vi "Memory Location Update.vi"(7 "Memory In":refnum<k21>, 8 "Data Valid":bool=TRUE, 10 "Address":u16, 11 "Data":fxp<+/-,16,1>) -> ()   [LabVIEW 2011]
uses:
  <vilib>/rvi/FXPMathLib/FxpConvert/subVIs/nifxpmath_Convert_SimConfig.ctl
  <vilib>/fxp/LVFixedPointQuantizationPolicyTypeDef.ctl
  <vilib>/fxp/LVFixedPointOverflowPolicyTypeDef.ctl
  <vilib>/rvi/FXPMathLib/basic elements/DSP48E/simVIs/niFpgaDsp48eRegisters.ctl
  <vilib>/rvi/FXPMathLib/basic elements/DSP48E/simVIs/niFpgaDsp48eEnables.ctl
  <vilib>/rvi/FXPMathLib/basic elements/DSP48E/simVIs/niFpgaDsp48eResets.ctl
  <vilib>/rvi/FXPMathLib/basic elements/DSP48E/simVIs/niFpgaDsp48eSimulationState.ctl
  <vilib>/rvi/FXPMathLib/basic elements/DSP48E/subVIs/niFpgaDsp48eType.ctl
  <vilib>/rvi/FXPMathLib/basic elements/DSP48E/subVIs/niFpgaDsp48eAlumodeOpmodeCarryinselState.ctl
  <vilib>/rvi/FXPMathLib/basic elements/DSP48E/subVIs/niFpgaDsp48eUseMultiplierState.ctl
  <vilib>/rvi/FXPMathLib/basic elements/DSP48E/subVIs/niFpgaDsp48eLogicUnitModeState.ctl
  <vilib>/rvi/FXPMathLib/basic elements/DSP48E/subVIs/niFpgaDsp48eSelectPatternState.ctl
  <vilib>/rvi/FXPMathLib/basic elements/DSP48E/subVIs/niFpgaDsp48eSelectMaskState.ctl
  <vilib>/rvi/FXPMathLib/basic elements/DSP48E/subVIs/niFpgaDsp48eAutoresetState.ctl
  <vilib>/rvi/FXPMathLib/FxpConvert/simVIs/DllFxpConvertTemp_sub.vi
  <vilib>/rvi/FXPMathLib/basic elements/DSP48E/simVIs/niFpgaDsp48eSimMultiplier.vi
  <vilib>/rvi/FXPMathLib/basic elements/DSP48E/simVIs/niFpgaDsp48eSimArithmetic.vi
  <vilib>/rvi/FXPMathLib/basic elements/DSP48E/simVIs/niFpgaDsp48eSimPatternDetect.vi
  <vilib>/rvi/FXPMathLib/basic elements/DSP48E/simVIs/niFpgaDsp48eSimP.vi
  <vilib>/rvi/FXPMathLib/basic elements/DSP48E/simVIs/niFpgaDsp48eSimUpdateState.vi
  <vilib>/rvi/FXPMathLib/basic elements/DSP48E/simVIs/niFpgaDsp48eCheckMode.vi
  <vilib>/rvi/FXPMathLib/basic elements/DSP48E/simVIs/niFpgaDsp48eReportInvalidMode.vi
  <vilib>/rvi/DataTransferAndStorage/Container/Common/niFpgaContainerExecOnDevCompGetState.vi
  <vilib>/rvi/Memory/Memory_Emulation/niFpgaMemoryEmulationValidateCache.vi
  <vilib>/rvi/DataTransferAndStorage/Container/Common/niFpgaContainerGetUniqueNameForEmu.vi
  <vilib>/rvi/Memory/Memory_Emulation/nirvimemoryEmulationManagerCache_InsertValue.vi
  <vilib>/Utility/error.llb/Clear Errors.vi
  <vilib>/rvi/Memory/Memory_Emulation/nirvimemoryEmulationManagerCache_GetValue.vi
  <vilib>/rvi/Memory/Memory_Emulation/nirvimemoryEmulationManagerCache_SetValue.vi
  <vilib>/rvi/FXPMathLib/FxpConvert/XNode/nifxpmath_Convert.xnode
  <vilib>/rvi/FXPMathLib/basic elements/DSP48E/XNode/niFpgaDsp48e.xnode
  <vilib>/rvi/FXPMathLib/basic elements/FxpDiscreteDelay/XNode/nifxpmath_DiscreteDelay.xnode
  <vilib>/rvi/DataTransferAndStorage/Container/XNode/niFpgaContainer.xnode
  <vilib>/rvi/Memory/Memory_Emulation/niFpgaMemoryEmulationRefIn.vi
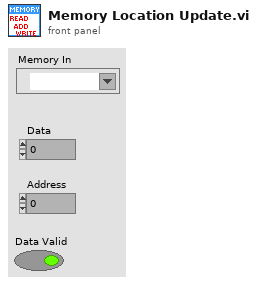
[diagram p1: front panel]
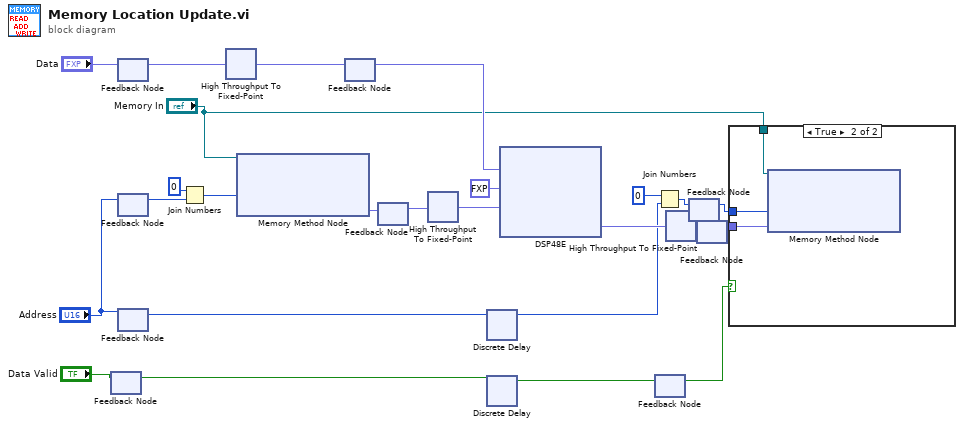
[diagram p0: block diagram]
diagram:
  n1 = feedback #1() -> (w8:bool)  [unwired: 1 in]
  n2 = feedback-in #1("Data Valid") -> ()
  n3 = feedback #2() -> (w13:fxp<+/-,16,1>)  [unwired: 1 in]
  n4 = feedback-in #2("Data") -> ()
  n5 = feedback #3() -> (w20:u16)  [unwired: 1 in]
  n6 = feedback-in #3("Address") -> ()
  n7 = feedback #4() -> (w11:u16)  [unwired: 1 in]
  n8 = feedback-in #4("Address") -> ()
  n9 = Join Numbers(hi=u16 0, lo=w20) -> ((hi.lo)=w6:u32)
  n10 = xnode "High Throughput To Fixed-Point"("x"=w13) -> ("y"=w12:fxp<+/-,30,1>)
  n11 = xnode ("Memory Method Node")("Address"=w6, "Memory In"="Memory In") -> ("Data"=w5:fxp<+/-,24,2>)  [unwired: 1 out]
  n12 = feedback #5() -> (w17:fxp<+/-,30,1>)  [unwired: 1 in]
  n13 = feedback-in #5(w12) -> ()
  n14 = feedback #6() -> (w15:fxp<+/-,24,2>)  [unwired: 1 in]
  n15 = feedback-in #6(w5) -> ()
  n16 = xnode "High Throughput To Fixed-Point"("x"=w15) -> ("y"=w14:fxp<+/-,48,2>)
  n17 = xnode "Discrete Delay"("D"=w11) -> ("Q"=w10:u16)
  n18 = xnode "Discrete Delay"("D"=w8) -> ("Q"=w7:bool)
  n19 = xnode "DSP48E"("a"=w17, "b"=fxp<+/-,18,18> 0.0, "c"=w14) -> ("p"=w23:fxp<+/-,48,2>)
  n20 = Join Numbers(hi=u16 0 ("lo"), lo=w10) -> ((hi.lo)=w22:u32)
  n21 = feedback-in #7(w7) -> ()
  n22 = feedback #7() -> (w1:bool)  [unwired: 1 in]
  n23 = xnode "High Throughput To Fixed-Point"("x"=w23) -> ("y"=w16:fxp<+/-,24,2>)
  n24 = feedback-in #8(w22) -> ()
  n25 = feedback #8() -> (w3:u32)  [unwired: 1 in]
  n26 = feedback-in #9(w16) -> ()
  n27 = feedback #9() -> (w2:fxp<+/-,24,2>)  [unwired: 1 in]
  n28 = case shown="True" w1 {
    tunnel: w3 -> [_ w28]
    tunnel: w2 -> [_ w27]
    tunnel: "Memory In" -> [_ w26]
    frame False {
    }
    frame True {
      n29 = xnode ("Memory Method Node")("Address"=w28, "Data"=w27, "Memory In"=w26) -> ()  [unwired: 1 out]
    }
  }
